vi "Configure AC Voltage.vi"(0 "VISA resource name":refnum<visa-resource-name>, 1 "Aperture Seconds":dbl, 2 "Bandwidth (30)":u16(ring) items=["3", "30", "300"], 3 "Unit":u16(ring) items=["Volt", "DB"], 5 "Auto Range? (T: Auto)":bool, 7 "Manual Range":dbl=10.0, 9 "Set Aperture or NPLC":bool=TRUE, 11 "error in (no error)":errorcluster, 12 "NPLC":dbl=1.0, 13 "DB Reference":dbl=1.0 min=1e-07 max=1000.0) -> (4 "VISA resource name out":refnum<visa-resource-name>, 15 "error out":errorcluster)   [LabVIEW 2025, in "Keithley DMM7510.lvlib"]
doc: "This VI configures the AC Voltage measurement and the related parameters."
uses:
  Keithley DMM7510.lvlib
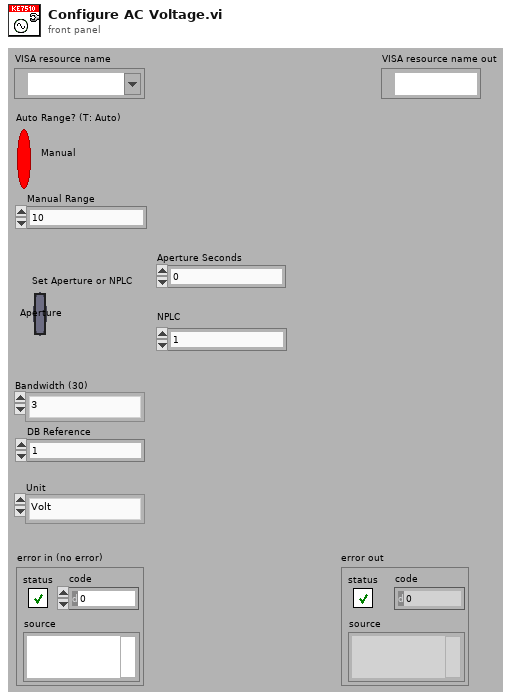
[diagram p1: front panel]
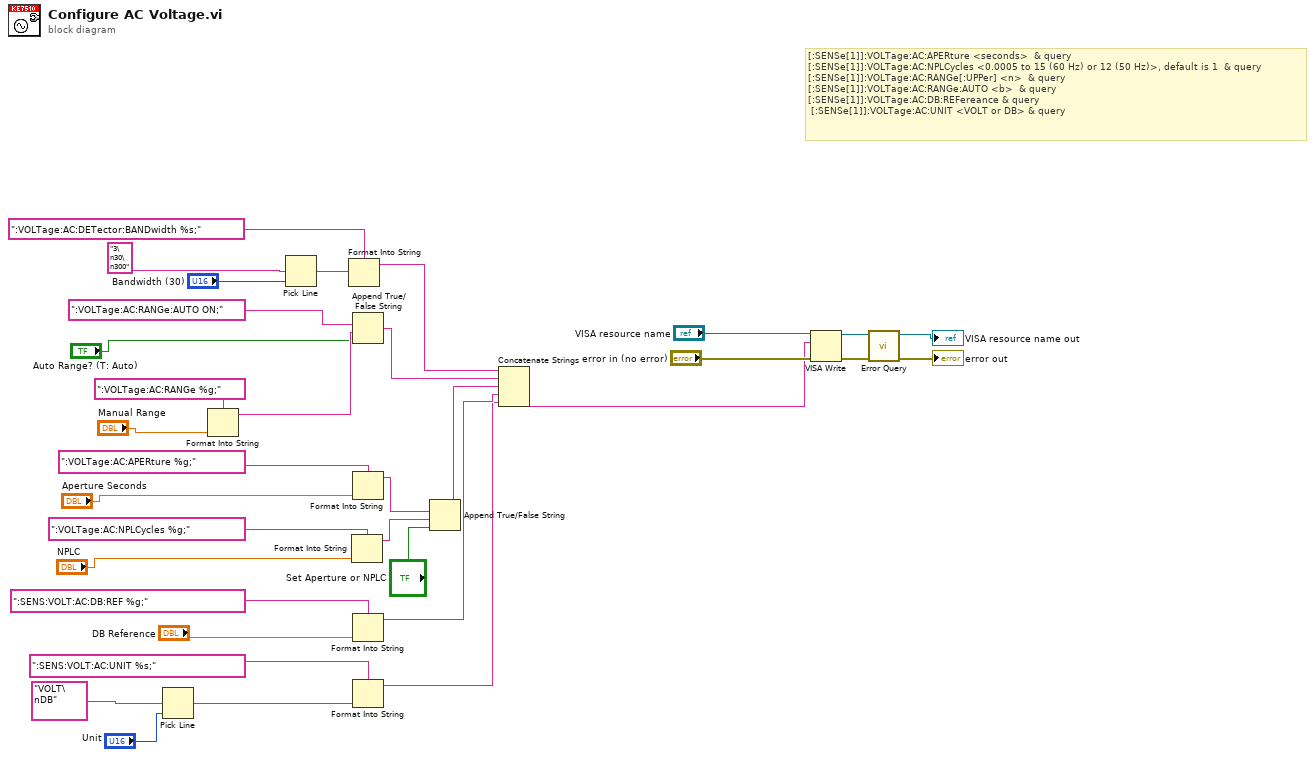
[diagram p0: block diagram]
diagram:
  # "[:SENSe[1]]:VOLTage:AC:APERture <seconds>  & query\n[:SENSe[1]]:VOLTage:AC:NPLCycles <0.0005 to 15 (60 Hz) or 12 (50 Hz)>, default is 1  & query\n[:SENSe[1]]:VOLTage:AC:RANGe[:UPPer] <n>  & query\n[:SENSe[1]]:VOLTage:AC:RANGe:AUTO <b>  & query\n[:SENSe[1]]:VOLTage:AC:DB:REFereance & query\n [:SENSe[1]]:VOLTage:AC:UNIT <VOLT or DB> & query"
  n1 = Pick Line(multi-line string="VOLT\nDB", line index="Unit") -> (output string=w19:string)  [unwired: 1 in]
  n2 = Format Into String(format string=":VOLTage:AC:RANGe %g;", "Manual Range") -> (resulting string=w29:string)  [unwired: 2 in, 1 out]
  n3 = Pick Line(multi-line string="3\n30\n300", line index="Bandwidth (30)") -> (output string=w10:string)  [unwired: 1 in]
  n4 = Format Into String(format string=":VOLTage:AC:DETector:BANDwidth %s;", w10) -> (resulting string=w26:string)  [unwired: 2 in, 1 out]
  n5 = Format Into String(format string=":VOLTage:AC:NPLCycles %g;", "NPLC") -> (resulting string=w2:string)  [unwired: 2 in, 1 out]
  n6 = Append True/False String(1:"Auto Range? (T: Auto)", 2:w29, 3:":VOLTage:AC:RANGe:AUTO ON;") -> (0:w25:string)  [unwired: 1 in]
  n7 = Format Into String(format string=":VOLTage:AC:APERture %g;", "Aperture Seconds") -> (resulting string=w3:string)  [unwired: 2 in, 1 out]
  n8 = Format Into String(format string=":SENS:VOLT:AC:DB:REF %g;", "DB Reference") -> (resulting string=w17:string)  [unwired: 2 in, 1 out]
  n9 = Format Into String(format string=":SENS:VOLT:AC:UNIT %s;", w19) -> (resulting string=w16:string)  [unwired: 2 in, 1 out]
  n10 = Append True/False String(1:"Set Aperture or NPLC", 2:w2, 3:w3) -> (0:w1:string)  [unwired: 1 in]
  n11 = Concatenate Strings(w26, w25, w1, w17, w16) -> (w24:string)
  n12 = VISA Write(VISA resource name="VISA resource name", write buffer=w24, error in (no error)="error in (no error)") -> (VISA resource name out=w15:refnum<visa-resource-name>, error out=w14:errorcluster)  [unwired: 1 out]
  n13 = call "Error Query.vi"("error in (no error)"=w14, "VISA resource name"=w15) -> ("error out"=→"error out":errorcluster, "VISA resource name out"=→"VISA resource name out":refnum<visa-resource-name>)  [unwired: 6 in, 2 out]
